vi "test variant to json null.vi"(8 "error in (no error)":errorcluster) -> (0 "error out":errorcluster)   [LabVIEW 2019, in "labview_json_tests.lvlib"]
uses:
  labview_json_tests.lvlib
  lib/labview_json.lvlib
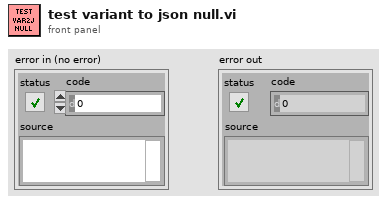
[diagram p1: front panel]
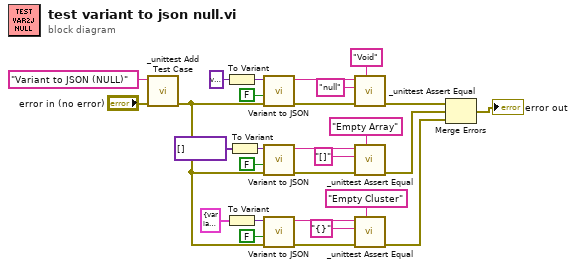
[diagram p0: block diagram]
diagram:
  n1 = call "_unittest Add Test Case.vi"("error in (no error)"="error in (no error)", "Test Case"="Variant to JSON (NULL)") -> ("error out"=w2:errorcluster)  [unwired: 9 in]
  n2 = To Variant(anything=variant) -> (Variant=w21:variant)
  n3 = To Variant(anything=cluster{variant} {variant}) -> (Variant=w8:variant)
  n4 = To Variant(anything=variant[] []) -> (Variant=w17:variant)
  n5 = call "Variant to JSON.vi"("error in (no error)"=w2, "Pretty Print? (F)"=FALSE, "Variant in"=w21) -> ("error out"=w24:errorcluster, "JSON"=w25:string)  [unwired: 7 in]
  n6 = call "Variant to JSON.vi"("error in (no error)"=w2, "Pretty Print? (F)"=FALSE, "Variant in"=w17) -> ("error out"=w14:errorcluster, "JSON"=w13:string)  [unwired: 7 in]
  n7 = call "Variant to JSON.vi"("error in (no error)"=w2, "Pretty Print? (F)"=FALSE, "Variant in"=w8) -> ("error out"=w6:errorcluster, "JSON"=w5:string)  [unwired: 7 in]
  n8 = call "_unittest Assert Equal.vi"("Message"="Void", "error in (no error)"=w24, "Expected Value"="null", "Actual Value"=w25) -> ("error out"=w20:errorcluster)  [unwired: 7 in]
  n9 = call "_unittest Assert Equal.vi"("Message"="Empty Array", "error in (no error)"=w14, "Expected Value"="[]", "Actual Value"=w13) -> ("error out"=w10:errorcluster)  [unwired: 7 in]
  n10 = call "_unittest Assert Equal.vi"("Message"="Empty Cluster", "error in (no error)"=w6, "Expected Value"="{}", "Actual Value"=w5) -> ("error out"=w3:errorcluster)  [unwired: 7 in]
  n11 = Merge Errors(w20, w10, w3) -> (→"error out":errorcluster)
